vi "UHR-Fleezers Control (host) - 10.5.vi"() -> ()   [LabVIEW 2011] (continued)
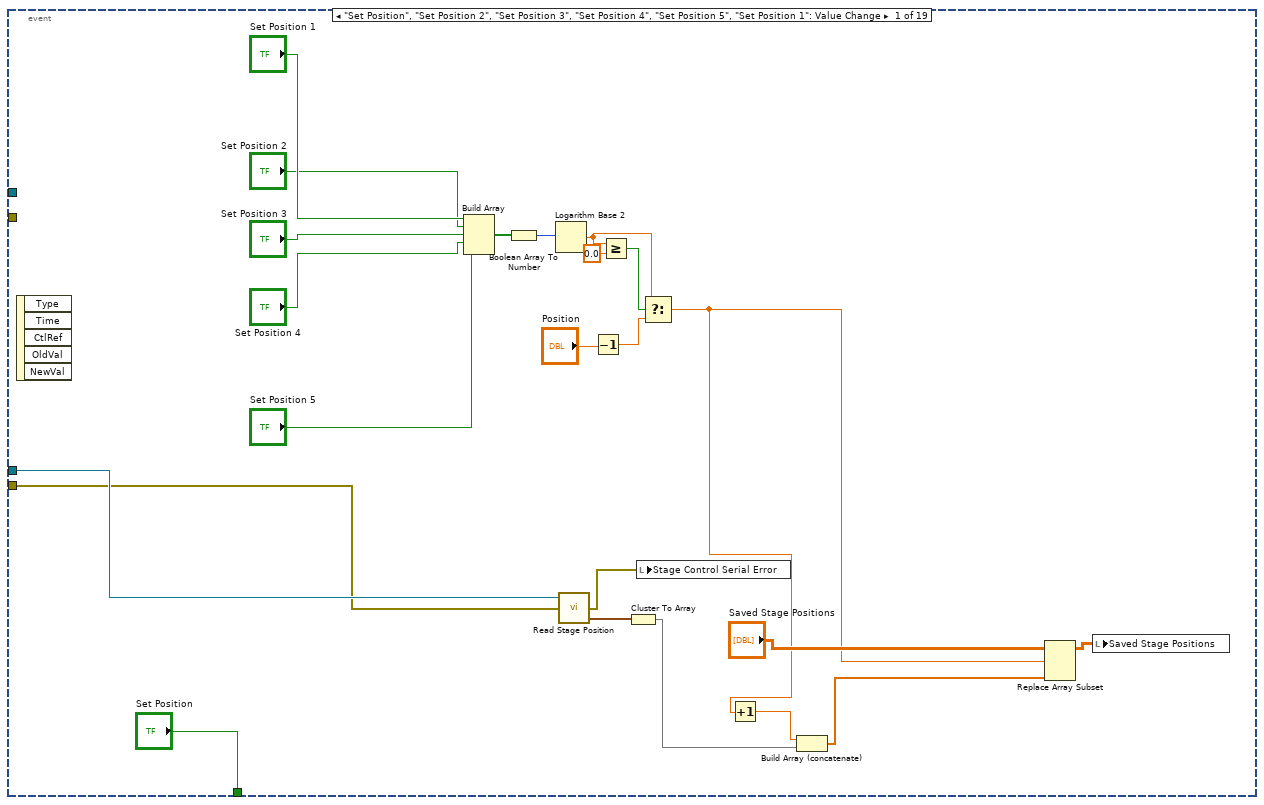
[diagram p2: hidden frame]
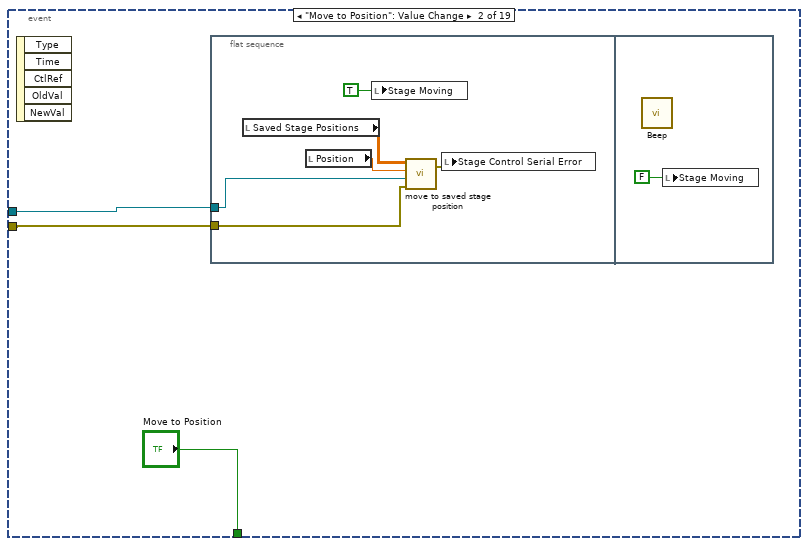
[diagram p3: hidden frame]
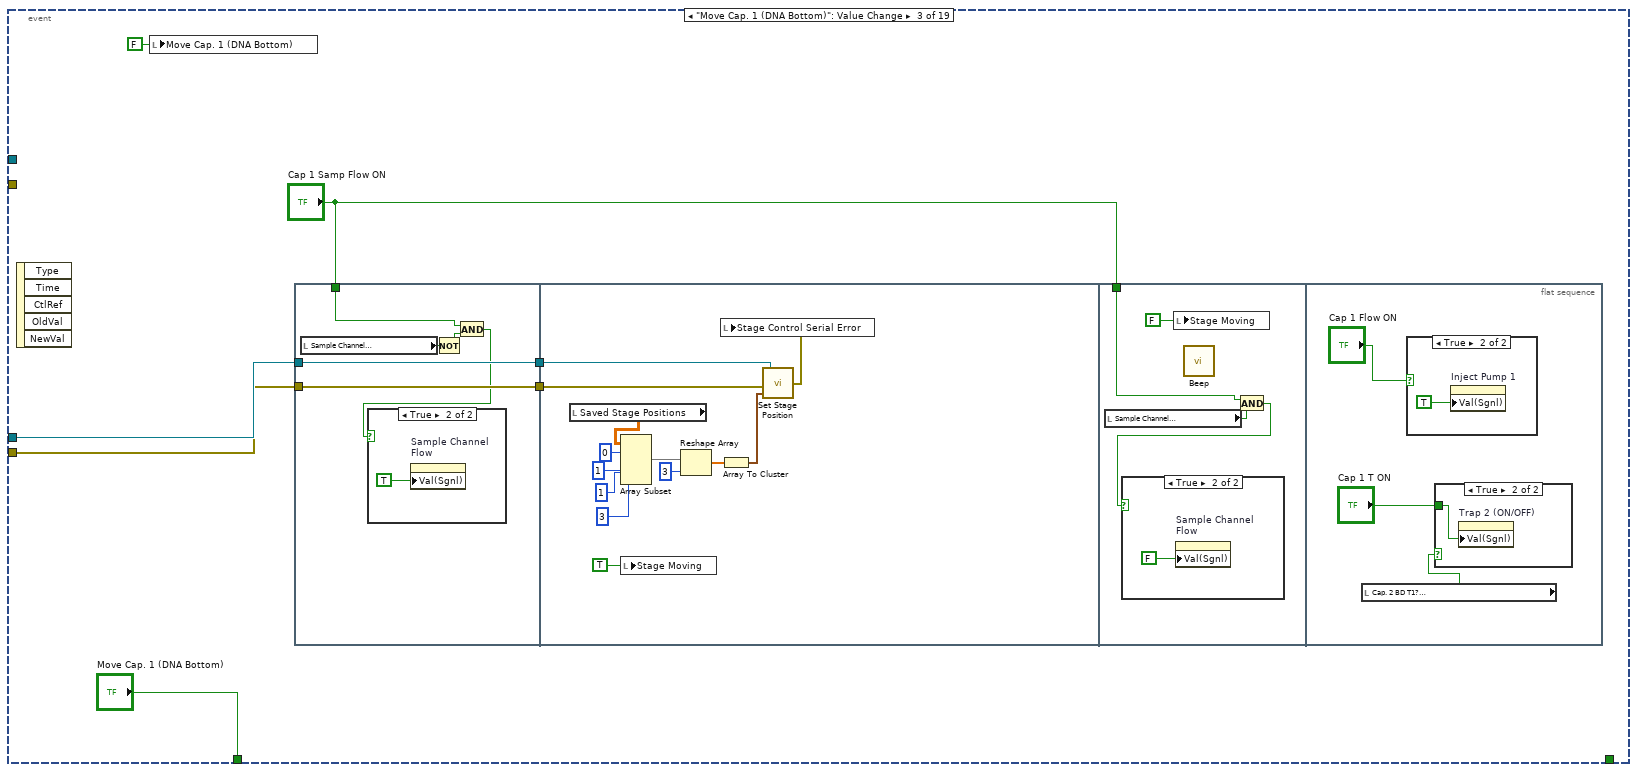
[diagram p4: hidden frame]
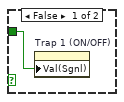
[diagram p8: hidden frame]
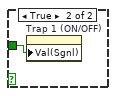
[diagram p12: hidden frame]
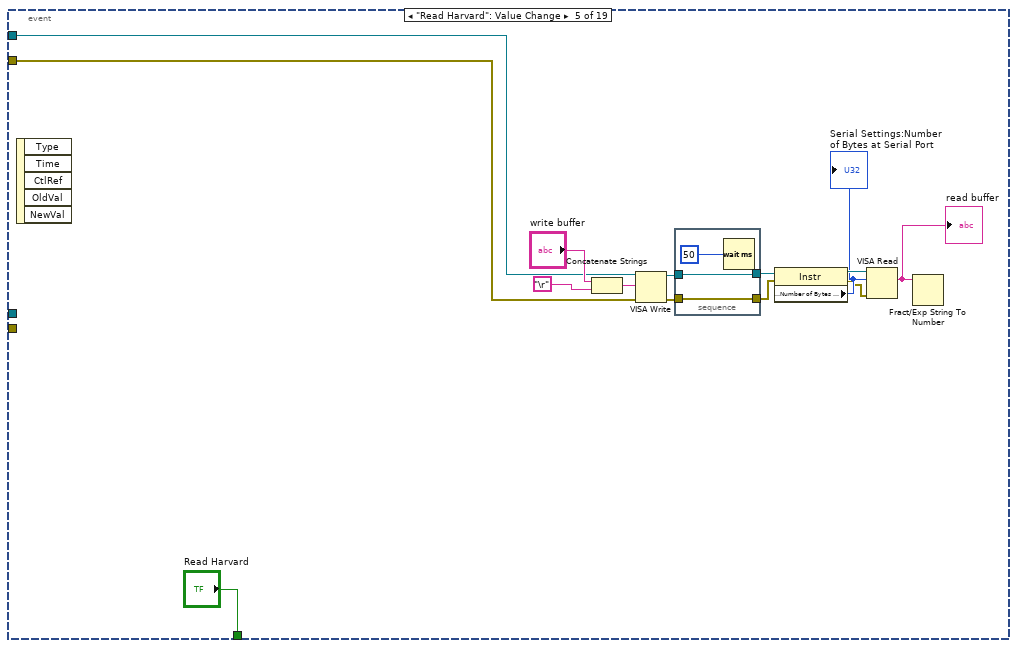
[diagram p13: hidden frame]
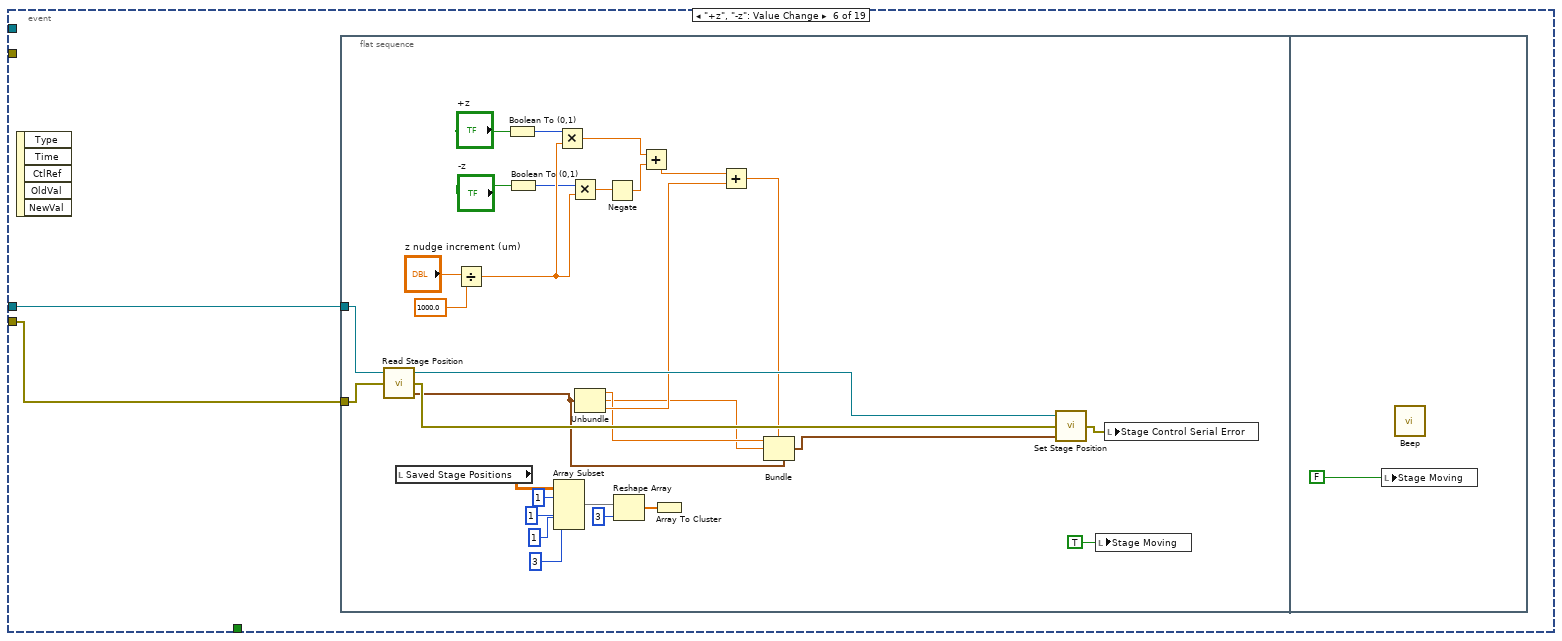
[diagram p14: hidden frame]
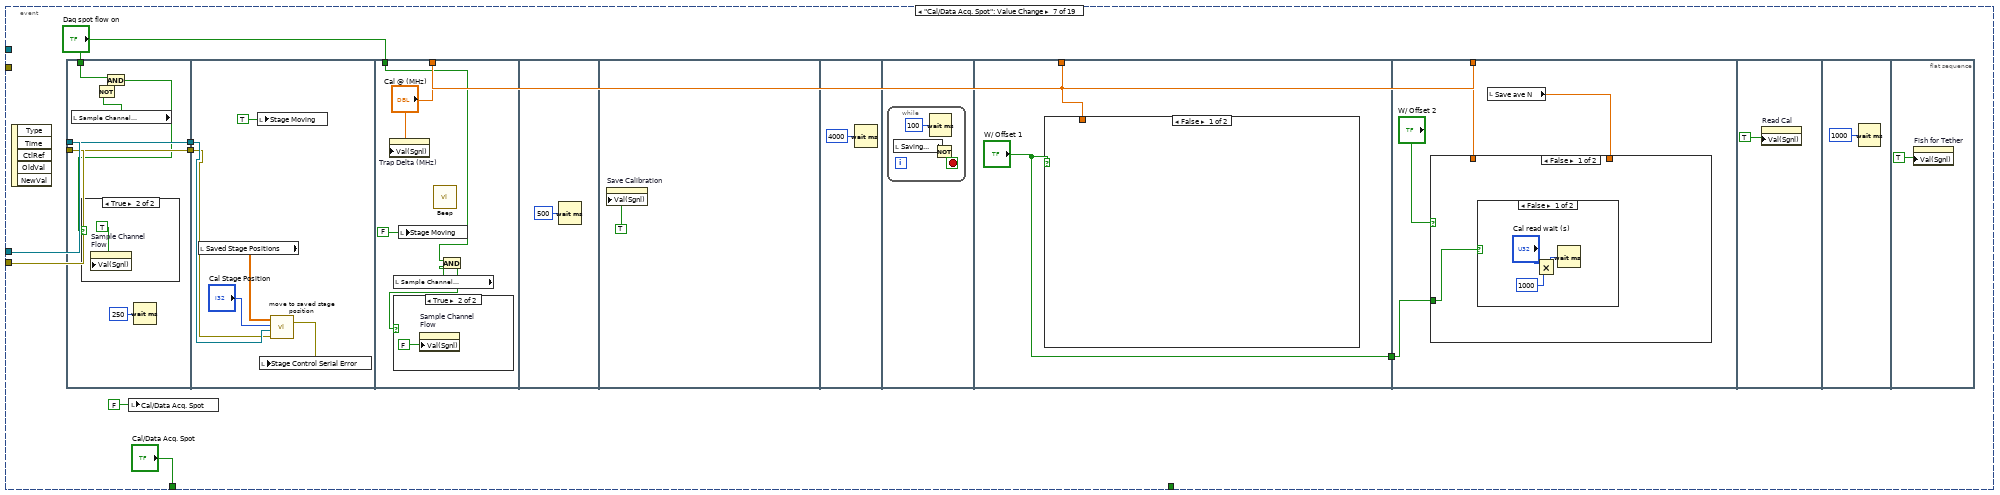
[diagram p15: hidden frame]
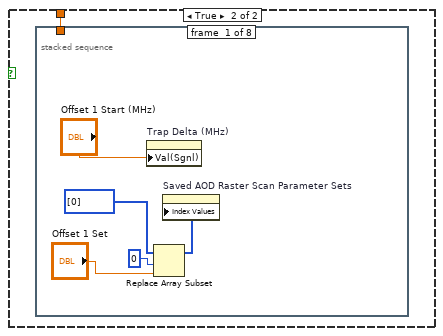
[diagram p18: hidden frame]
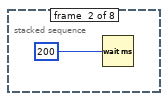
[diagram p19: hidden frame]
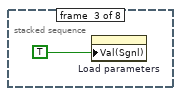
[diagram p20: hidden frame]
    n2214 = Subtract(x=w2595, y="Offset (nm)") -> (x-y=w2773:dbl[])
    n2215 = case shown="True" "Read Lateness and Rel Phase" {
      tunnel: w2615 -> [w3099 w3121]
      tunnel: w2614 -> [w3100 w3120]
      tunnel: [w3099 w3119] -> w2802
      tunnel: [w3100 w3118] -> w2801
      frame False {
      }
      frame True {
        n2216 = xnode "Read/Write Control"("FPGA VI Reference In"=w3121, "error in"=w3120) -> ("FPGA VI Reference Out"=w3119:T19, "error out"=w3118:errorcluster, "GI Relative phase"=→"GI relative phase":i16, "Relative phase"=→"Relative phase (AI1)":i16, "AI Late Counter"=→"Late Counter (AI1)":u16, "GI Late Counter"=→"GI Late Counter":u16, "MCL Late Counter"=→"MCL Late Counter":u16, "MCL Relative Phase"=→"Relative Phase (MCL)":i16, "APD Acq Relative Phase"=→"APD Acq Relative Phase":i16, "APD 1 Gate Relative Phase"=→"APD 1 Gate Relative Phase":i16, "APD 2 Gate Relative Phase"=→"APD 2 Gate Relative Phase":i16, "APD Acq Late Counter"=→"APD Acq Late Counter":u16, "APD 1 Gate Late Counter"=→"APD 1 Gate Late Counter":u16, "APD 2 Gate Late Counter"=→"APD 2 Gate Late Counter":u16, "Green FB Relative Phase"=→"Relative phase (Green FB)":i16, "GI Relative phase 2"=→"GI relative phase 2":i16, "GI Late Counter 2"=→"GI Late Counter 2":u16, "Trap Pos FIFO Timeout"=→"Trap Pos FIFO Timeout":u16, "Trap AI FIFO Timeout"=→"Trap AI FIFO Timeout":u16)
      }
    }
    n2217 = call <vilib>:"Mean.vi"("X"=w2775) -> ("mean"=w2601:dbl)  [unwired: 1 out]
    "T2 X" <- w2601
    n2218 = Negate(x=w2775) -> (-x=w2776:dbl[])
    n2219 = call <vilib>:"Mean.vi"("X"=w2599) -> ("mean"=w2602:dbl)  [unwired: 1 out]
    "T1 X" <- w2602
    n2220 = Negate(x=w2601) -> (-x=w2600:dbl)
    n2221 = Bundle By Name(cluster=w2808, "Y"=w2773) -> (w2747:waveform(dbl))
    "Bead Separation" <- w2747
    n2222 = Add(x=w2599, y=w2776) -> (x+y=w2777:dbl[])
    n2223 = Add(x=w2602, y=w2600) -> (x+y=w2824:dbl)
    n2224 = Subtract(x=w2602, y=w2600) -> (x-y=→"Difference":dbl)
    n2225 = Divide(x=w2777, y=2.0) -> (x/y=→"Vec Mean of T1 T2":dbl[])
    n2226 = Divide(x=w2824, y=2.0) -> (x/y=w2779:dbl)
    "Mean" <- w2779
    n2227 = feedback-in #21("Trap Trig. Fl.") -> ()
    n2228 = feedback #21("Trap Trig. Fl.") -> (w2633:bool)
    n2229 = And(x=w2635, y=w2633) -> (x .and. y?=w2634:bool)
    n2230 = case "If have just turned off triggering" shown="True" w2634 {
      tunnel: w2615 -> [_ w2934]
      tunnel: w2614 -> [_ w2933]
      frame False {
      }
      frame True {
        w2932 = FALSE ("FPGA Trap Trig")
        n2231 = xnode "Read/Write Control"("FPGA VI Reference In"=w2934, "error in"=w2933, "FPGA Trap Trig"=w2932) -> ("FPGA VI Reference Out"=w2931:T19, "error out"=w2930:errorcluster)
        n2232 = xnode "Read/Write Control"("FPGA VI Reference In"=w2931, "error in"=w2930, "TTrig?"=w2932) -> ()  [unwired: 2 out]
        n2233 = local write "Initializing"(FALSE ("Initializing")) -> ()
        n2234 = local write "Triggered"(FALSE ("Triggered")) -> ()
        n2235 = local write "Waiting"(FALSE ("Waiting")) -> ()
      }
    }
    n2236 = Not(x=w2633) -> (.not. x?=w2646:bool)
    n2237 = And(x="Trap Trig. Fl.", y=w2646) -> (x .and. y?=w2643:bool)
    n2238 = local read "Tether"() -> (w2780:bool)
    n2239 = Or(x=w2643, y="Reinitialize") -> (x .or. y?=w2629:bool)
    n2240 = feedback #22(w2639) -> (w2644:string)
    n2241 = Select(t=w2639, s=w2643, f=w2644) -> (s? t:f=w2638:string)
    n2242 = Select(t=w2639, s="Reinitialize", f=w2638) -> (s? t:f=w2637:string)
    n2243 = feedback #23(0) -> (w2641:i32)
    n2244 = feedback #24(w2773) -> (w2772:dbl[])
    n2245 = Build Array (concatenate)(w2773, w2772) -> (w2596:dbl[])
    n2246 = case "For determining if there is a tether still" shown="True" w2780 {
      tunnel: w2779 -> [_ w3058]
      frame False {
      }
      frame True {
        n2247 = Greater?(x="Lost Tether Alarm Threshold (pN)", y=w3058) -> (0:w3056:bool)
        n2248 = case shown="True" w3056 {
          frame False {
          }
          frame True {
            w3059 = FALSE ("Value (Signaling)")
            n2249 = flat-sequence {
              frame #0 {
                # "stop only if saving"
                n2250 = local read "Saving..."() -> (w3071:bool)
                n2251 = And(x=w3071, y="TA Cancel Save?") -> (x .and. y?=w3070:bool)
                n2252 = local write "Stop Saving"(w3070) -> ()
              }
              frame #1 {
                n2253 = case shown="True" "TA Green Off?" {
                  frame False {
                  }
                  frame True {
                    w3074 = FALSE ("Fl. Triggered...")
                    n2254 = local write "Fl. Triggered..."(w3074) -> ()
                    n2255 = property on="Green Laser ON/Interlacing" class="Bool (strict)"("Val(Sgnl)"=w3074) -> ()  [unwired: 2 in, 2 out]
                  }
                }
              }
            }
            n2256 = local read "Time tether formed"() -> (w3065:timestamp)
            n2257 = Get Date/Time In Seconds() -> (seconds since 1Jan1904=w3066:timestamp)
            n2258 = Subtract(x=w3066, y=w3065) -> (x-y=w3064:dbl)
            n2259 = Number To Decimal String(number=w3064) -> (decimal integer string=w3061:string)  [unwired: 1 out]
            n2260 = local read "Messages"() -> (w3068:string)
            n2261 = call <vilib>:"Beep.vi"() -> ()  [unwired: 3 in, 9 out]
            n2262 = Concatenate Strings("Lost tether (" ("Message to add"), w3061, " s)." ("string")) -> (w3063:string)
            n2263 = local write "Tether"(FALSE ("Tether")) -> ()
            n2264 = call "Update messages.vi"("Message to add"=w3063, "Old message string"=w3068) -> ("New message string"=w3067:string)
            n2265 = local write "Messages"(w3067) -> ()
            n2266 = local write "Dip for Protein"(w3059) -> ()
            n2267 = property on="Trap Pos. FB ON" class="Bool (strict)"("Val(Sgnl)"=w3059) -> ()  [unwired: 2 in, 2 out]
            n2268 = property on="Trap Trig. Fl." class="Bool (strict)"("Val(Sgnl)"=w3059) -> ()  [unwired: 2 in, 2 out]
          }
        }
      }
    }
    n2269 = case "For triggering actions based on the trap position (e.g., turning the excitation laser on if trap under feedback moves so far)" shown="True" "Trap Trig. Fl." {
      tunnel: w2624 -> [_ w2947]
      tunnel: w2637 -> [_ w2946]
      tunnel: ["" ("t") w2945] -> w2645
      tunnel: w2629 -> [_ w2944]
      tunnel: [0 ("t") w2943] -> w2642
      tunnel: w2641 -> [_ w2942]
      tunnel: w2615 -> [_ w2941]
      tunnel: w2614 -> [_ w2940]
      frame False {
      }
      frame True {
        n2270 = case shown="\"Initialize\", Default" w2946 {
          tunnel: w2947 -> [w2964 _ _ w3012]
          tunnel: [w2961 w2993 "" ("t") w3015] -> w2945
          tunnel: w2944 -> [_ _ _ w3003]
          tunnel: [w2960 w2990 0 ("t") w3004] -> w2943
          tunnel: w2942 -> [_ w2992 _ w3010]
          tunnel: w2941 -> [w2949 w2987 _ w3006]
          tunnel: w2940 -> [w2948 w2986 _ w3005]
          frame "Wait for trigger" {
            n2271 = local read "Trap Trig. (FPGA)"() -> (w2952:bool)
            n2272 = Subtract(x=w2964, y="Mean T1 Position\nto compare (nm)") -> (x-y=w2957:dbl[])
            n2273 = call <vilib>:"Std Deviation and Variance.vi"("X"=w2957) -> ("mean"=→"mean":dbl, "standard deviation"=→"standard\ndeviation":dbl)  [unwired: 1 in, 1 out]
            n2274 = Array Max & Min(array=w2957) -> (max value=→"max value":dbl, min value=→"min value":dbl)  [unwired: 2 out]
            n2275 = Greater?(x=w2957, y="Threshold (nm)") -> (0:w2967:bool[])
            n2276 = case shown="True" w2952 {
              tunnel: w2949 -> [_ w2973]
              tunnel: w2948 -> [_ w2972]
              tunnel: [FALSE ("TTrig?") w2971] -> w2955
              frame False {
              }
              frame True {
                n2277 = xnode "Read/Write Control"("FPGA VI Reference In"=w2973, "error in"=w2972) -> ("TTrig?"=w2971:bool)  [unwired: 2 out]
              }
            }
            n2278 = Or Array Elements(Boolean array=w2967) -> (logical OR=w2954:bool)
            n2279 = Select(t=w2955, s=w2952, f=w2954) -> (s? t:f=w2953:bool)
            n2280 = Not(x=w2952) -> (.not. x?=w2951:bool)
            n2281 = And(x=w2953, y=w2951) -> (x .and. y?=w2950:bool)
            n2282 = Select(t="Triggered", s=w2953, f="Wait for trigger") -> (s? t:f=w2961:string)
            n2283 = case shown="True" w2953 {
              tunnel: [0 0] -> w2960
              tunnel: w2949 -> [_ w2978]
              tunnel: w2948 -> [_ w2977]
              frame False {
                "Waiting" <- TRUE ("Waiting")
              }
              frame True {
                n2284 = xnode "Read/Write Control"("FPGA VI Reference In"=w2978, "error in"=w2977, "TTrig?"=FALSE) -> ()  [unwired: 2 out]
                n2285 = local read "Messages"() -> (w2981:string)
                n2286 = call <vilib>:"Beep.vi"() -> ()  [unwired: 12 in]
                n2287 = call "Update messages.vi"("Message to add"="Unwinding trigger.", "Old message string"=w2981) -> ("New message string"=w2982:string)
                n2288 = local write "Messages"(w2982) -> ()
                n2289 = local write "Waiting"(FALSE ("Waiting")) -> ()
                "Triggered" <- TRUE ("Triggered")
              }
            }
            n2290 = case "Only need to turn on laser if host triggered" shown="True" w2950 {
              frame False {
              }
              frame True {
                n2291 = property on="Green Laser ON/Interlacing" class="Bool (strict)"("Val(Sgnl)"=TRUE ("Value (Signaling)")) -> ()  [unwired: 2 in, 2 out]
              }
            }
          }
          frame "Triggered" {
            n2292 = local read "Trap Trig. (FPGA)"() -> (w2989:bool)
            n2293 = Increment(x=w2992) -> (x+1=w2990:i32)
            n2294 = Greater Or Equal?(x=w2990, y="Fl. ON time (n)") -> (x >= y?=w2988:bool)
            n2295 = Select(t="Wait for trigger", s=w2988, f="Triggered" ("t")) -> (s? t:f=w2993:string)
            n2296 = And(x=w2988, y=w2989) -> (x .and. y?=w2985:bool)
            n2297 = case shown="True" w2985 {
              tunnel: w2987 -> [_ w2997]
              tunnel: w2986 -> [_ w2996]
              frame False {
              }
              frame True {
                n2298 = xnode "Read/Write Control"("FPGA VI Reference In"=w2997, "error in"=w2996, "FPGA Trap Trig"=TRUE) -> ()  [unwired: 2 out]
              }
            }
            n2299 = case shown="True" w2988 {
              frame False {
              }
              frame True {
                w2999 = FALSE ("Value (Signaling)")
                n2300 = local write "Triggered"(w2999) -> ()
                n2301 = local write "Waiting"(TRUE ("Waiting")) -> ()
                n2302 = property on="Green Laser ON/Interlacing" class="Bool (strict)"("Val(Sgnl)"=w2999) -> ()  [unwired: 2 in, 2 out]
              }
            }
          }
          frame "Do nothing" {
          }
          frame "Initialize", Default {
            n2303 = Increment(x=w3010) -> (x+1=w3014:i32)
            n2304 = Select(t=1, s=w3003, f=w3014) -> (s? t:f=w3004:i32)
            n2305 = feedback #25(w3012) -> (w3018:dbl[])
            n2306 = Build Array (concatenate)(w3012, w3018) -> (w3011:dbl[])
            n2307 = Greater Or Equal?(x=w3004, y="Wait to get offset (n)") -> (x >= y?=w3007:bool)
            n2308 = Select(t=w3012, s=w3003, f=w3011) -> (s? t:f=w3013:dbl[])
            n2309 = feedback-in #25(w3013) -> ()
            n2310 = call <vilib>:"Mean.vi"("X"=w3013) -> ("mean"=w3008:dbl)  [unwired: 1 out]
            n2311 = local write "Mean T1 Position\nto compare (nm)"(w3008) -> ()
            n2312 = case shown="True" w3003 {
              tunnel: w3006 -> [_ w3024]
              tunnel: w3005 -> [_ w3023]
              frame False {
              }
              frame True {
                w3020 = FALSE ("FPGA Trap Trig")
                n2313 = xnode "Read/Write Control"("FPGA VI Reference In"=w3024, "error in"=w3023, "FPGA Trap Trig"=w3020) -> ("FPGA VI Reference Out"=w3022:T19, "error out"=w3021:errorcluster)
                n2314 = xnode "Read/Write Control"("FPGA VI Reference In"=w3022, "error in"=w3021, "TTrig?"=w3020) -> ()  [unwired: 2 out]
              }
            }
            n2315 = Select(t="Wait for trigger", s=w3007, f="Initialize") -> (s? t:f=w3015:string)
            n2316 = case shown="True" w3007 {
              tunnel: w3008 -> [_ w3027]
              tunnel: w3006 -> [_ w3036]
              tunnel: w3005 -> [_ w3035]
              frame False {
                n2317 = local write "Waiting"(FALSE ("Waiting")) -> ()
                "Initializing" <- TRUE ("Initializing")
              }
              frame True {
                n2318 = local read "Threshold (nm)"() -> (w3039:dbl)
                n2319 = local read "AOM X Cal (nm/MHz)"() -> (w3038:dbl)
                n2320 = Add(x=w3027, y=w3039) -> (x+y=w3040:dbl)
                n2321 = Divide(x=w3040, y=w3038) -> (x/y=w3037:dbl)
                n2322 = call "IR AOM freq to word.vi"("Frequency In (MHz)"=w3037) -> ("Frequency Word Out (double)"=w3034:dbl)
                n2323 = local write "Initializing"(FALSE ("Initializing")) -> ()
                n2324 = local write "Waiting"(TRUE ("Waiting")) -> ()
                n2325 = To Quad Integer(1:w3034) -> (0:w3033:i64)
                n2326 = xnode "Read/Write Control"("FPGA VI Reference In"=w3036, "error in"=w3035, "FPGA TTrig Thresh"=w3033) -> ("FPGA VI Reference Out"=w3030:T19, "error out"=w3029:errorcluster)
                n2327 = xnode "Read/Write Control"("FPGA VI Reference In"=w3030, "error in"=w3029, "FPGA Trap Trig"=TRUE) -> ()  [unwired: 2 out]
              }
            }
          }
        }
      }
    }
    n2328 = feedback-in #22(w2645) -> ()
    n2329 = feedback-in #23(w2642) -> ()
    n2330 = Split 1D Array(array=w2596, index=w2659) -> (first subarray=w2769:dbl[])  [unwired: 1 out]
    n2331 = feedback-in #24(w2769) -> ()
    n2332 = call <vilib>:"Mean.vi"("X"=w2769) -> ("mean"=w2768:dbl)  [unwired: 1 out]
    "Bead Mean (nm)" <- w2768
    n2333 = Subtract(x=w2769, y=w2768) -> (x-y=w2767:dbl[])
    n2334 = Square(x=w2767) -> (x^2=w2766:dbl[])
    n2335 = call <vilib>:"Mean.vi"("X"=w2766) -> ("mean"=w2765:dbl)  [unwired: 1 out]
    n2336 = Square Root(x=w2765) -> (sqrt(x)=w2764:dbl)
    n2337 = Multiply(x=10.0, y=w2764) -> (x*y=→"RMS (Ang)":dbl)
    n2338 = xnode "Read/Write Control"("FPGA VI Reference In"=w2802, "error in"=w2801) -> ("FPGA VI Reference Out"=w2627:T19, "error out"=w2626:errorcluster, "AI2 Y Sum Set 1"=w2908:i16, "AI2 Y Sum Set 2"=w2907:i16, "AI1 X Set 1"=w2691:fxp<+/-,16,1>, "AI1 X Set 2"=w2690:fxp<+/-,16,1>, "Trap Pos FB Int Signal"=→"Trap Pos FB Int Signal":fxp<+/-,24,9>, "Trap Pos FB Int-Norm Signal"=→"Trap Pos FB Int-Norm Signal":fxp<+/-,16,1>, "Trap Pos FB Action"=w2684:i64, "Scanning"=→"AOD Scanning":bool, "Scan I"=→"AOD Scan I":u64, "Scanning MCL"=w2910:bool, "Scan I (MCL)"=→"MCL Scan I":u64, "Green FB Signals"=w2847:T46, "TTrig Sig"=w2613:i64, "TTrig Fin Thresh"=w2609:i64)
    "MCL Scanning" <- w2910
    "Trap Pos FB Action" <- w2684
    n2339 = local read "FB Trig Integrate"() -> (w2607:u32)
    n2340 = Divide(x=w2613, y=w2607) -> (x/y=w2606:dbl)
    "TTrig Sig (Int)" <- w2606
    n2341 = Divide(x=w2609, y=w2607) -> (x/y=w2604:dbl)
    "TTrig Fin Thresh (Int)" <- w2604
    n2342 = local read "AOM X Cal (nm/MHz)"() -> (w2612:dbl)
    n2343 = local read "AI2 (V)"() -> (w2909:cluster{"Set 1":dbl, "Set 2":dbl})
    n2344 = Bundle By Name(cluster=w2909, "Set 1"=w2908, "Set 2"=w2907) -> (w2905:cluster{"Set 1":dbl, "Set 2":dbl})
    n2345 = Divide(x=w2684, y=327.67) -> (x/y=→"Action (%)":dbl)
    n2346 = local read "Trap X (AI1)"() -> (w2704:T10)
    n2347 = call "IR AOM word double to freq.vi"("Frequency Word In (double)"=w2604) -> ("Frequency Out (MHz)"=w2603:dbl)
    n2348 = call "IR AOM word double to freq.vi"("Frequency Word In (double)"=w2606) -> ("Frequency Out (MHz)"=w2605:dbl)
    n2349 = Divide(x=w2905, y=3276.7) -> (x/y=w2904:cluster{"Set 1":dbl, "Set 2":dbl})
    n2350 = Multiply(x=w2605, y=w2612) -> (x*y=w2611:dbl)
    "TTrig Sig (nm)" <- w2611
    n2351 = Multiply(x=w2603, y=w2612) -> (x*y=w2610:dbl)
    "TTrig Fin Thresh (nm)" <- w2610
    n2352 = local write "AI2 (V)"(w2904) -> ()
    n2353 = Bundle(cluster=w2704, "Trap 1"=w2691, "Trap 2"=w2690) -> (→"Trap X (AI1)":T10)
    n2354 = Bundle(w2611, w2610) -> (→"TTrig":cluster{dbl, dbl})  [unwired: 1 in]
    n2355 = Divide(x=w2847, y=3276.7) -> (x/y=w2843:T47)
    n2356 = Unbundle By Name(w2843) -> ("Green FB Ch 0"=w2846:dbl, "Green FB Ch 1"=w2845:dbl, "Green FB Ch 2"=w2844:dbl)
    n2357 = Divide(x=w2846, y=w2844) -> (x/y=w2842:dbl)
    n2358 = Divide(x=w2845, y=w2844) -> (x/y=w2841:dbl)
    n2359 = flat-sequence "To save data" {
      tunnel: [w3895] -> w2928
      tunnel: [w3896] -> w2927
      tunnel: w2878 -> [w3889]
      tunnel: w2632 -> [w3893]
      tunnel: ["Save Calibration"] -> w2901
      tunnel: w2898 -> [w3892]
      tunnel: [w3885] -> w2897
      tunnel: [w3882] -> w2896
      tunnel: [w3879] -> w2895
      tunnel: w2877 -> [w3881]
      tunnel: w2784 -> [w3875]
      tunnel: [w3875] -> w2783
      tunnel: ["Start Saving"] -> w2749
      tunnel: [w3869] -> w2672
      tunnel: [w3868] -> w2671
      tunnel: w2928 -> [w4130]
      tunnel: w2927 -> [w4129]
      tunnel: w2673 -> [w4128]
      tunnel: w2901 -> [w4127]
      tunnel: w2897 -> [w4125]
      tunnel: w2896 -> [w4124]
      tunnel: w2895 -> [w4123]
      tunnel: w2758 -> [w4122]
      tunnel: w2794 -> [w4121]
      tunnel: w2783 -> [w4120]
      tunnel: w2749 -> [w4119]
      tunnel: w2747 -> [w4118]
      tunnel: w2723 -> [w4117]
      tunnel: w2672 -> [w4116]
      tunnel: w2671 -> [w4115]
      tunnel: w2670 -> [w4114]
      frame #0 {
        n2360 = Or(x="Save N Sets", y="Start Saving") -> (x .or. y?=w3876:bool)
        n2361 = To Double Precision Float(number=w3892) -> (double precision float=w3886:dbl)
        n2362 = Build Array(w3876, "Save Calibration", w3889, w3881) -> (w3891:bool[])
        n2363 = Compound Arithmetic op=OR("Save Calibration", w3889, w3876, w3881) -> (w3894:bool)
        n2364 = Boolean Array To Number(Boolean array=w3891) -> (number=w3888:u32)
        n2365 = feedback #26(FALSE ("Save APD Data\nwith Trap Data")) -> (w3870:bool)
        n2366 = feedback #27(refnum<k0> refnum) -> (w3897:refnum<file>)
        n2367 = feedback #28(refnum<k0> refnum) -> (w3872:refnum<file>)
        n2368 = feedback #29(FALSE ("Save APD Data\nwith Trap Data")) -> (w3880:bool)
        n2369 = feedback #30(refnum<k0> refnum) -> (w3883:refnum<file>)
        n2370 = feedback #31(0) -> (w3899:i32)
        n2371 = feedback #32() -> (w3887:u32)  [unwired: 1 out]
        n2372 = case shown="True" w3894 {
          tunnel: [w3906 1] -> w3895
          tunnel: w3899 -> [w3908 _]
          tunnel: [w3907 w3926] -> w3896
          tunnel: w3897 -> [w3907 _]
          tunnel: w3893 -> [_ w3946]
          tunnel: w3886 -> [_ w3944]
          tunnel: w3888 -> [_ w3947]
          tunnel: [w3905 w3925] -> w3885
          tunnel: w3887 -> [w3905 _]
          tunnel: [w3904 w3923] -> w3882
          tunnel: w3883 -> [w3904 _]
          tunnel: [w3903 w3922] -> w3879
          tunnel: w3880 -> [w3903 _]
          tunnel: "Start Saving" -> [_ w3920]
          tunnel: w3875 -> [_ w3919]
          tunnel: [w3902 w3910] -> w3868
          tunnel: w3872 -> [w3902 _]
          tunnel: [w3901 w3909] -> w3869
          tunnel: w3870 -> [w3901 _]
          frame False {
            n2373 = Increment(x=w3908) -> (x+1=w3906:i32)
          }
          frame True {
            w3916 = FALSE ("Start Saving")
            w3921 = 9.0  # File Version
            w3929 = FALSE ("prepend array or string size? (T)")
            w3927 = T24."big-endian, network order" ("byte order (0:big-endian, network order)")
            n2374 = local read "BD 1 Frequency 1 (MHz)"() -> (w3943:dbl)
            n2375 = local read "BD 2 Frequency 1 (MHz)"() -> (w3942:dbl)
            n2376 = local read "BD 1 Frequency 2 (MHz)"() -> (w3941:dbl)
            n2377 = local read "BD 2 Frequency 2 (MHz)"() -> (w3940:dbl)
            n2378 = local read "BD 1 Frequency 3 (MHz)"() -> (w3939:dbl)
            n2379 = local read "BD 2 Frequency 3 (MHz)"() -> (w3938:dbl)
            n2380 = Array Size(array=w3919) -> (size(s)=w3918:i32)
            n2381 = To Double Precision Float(number=w3918) -> (double precision float=w3917:dbl)
            n2382 = local write "Save Calibration"(w3916) -> ()
            n2383 = local write "Start Saving"(w3916) -> ()
            n2384 = Build Array("Save APD Data\nwith Trap Data", "Save Trap Pos. Data") -> (w3913:bool[])
            n2385 = Boolean Array To Number(Boolean array=w3913) -> (number=w3912:u32)
            n2386 = Build Array(w3943, w3942, w3941, w3940, w3939, w3938) -> (w3937:dbl[])
            n2387 = case shown="4" w3947 {
              tunnel: w3946 -> [w4018 w4038 w4054 w4092]
              tunnel: w3917 -> [w4023 w4045 w4074 w4111]
              tunnel: w3944 -> [w4022 w4044 w4073 w4110]
              tunnel: [w4019 w4040 w4065 w4102] -> w3935
              tunnel: [w4010 "Cal sets to save" w4055 w4093] -> w3925
              tunnel: w3937 -> [w4020 w4041 w4067 w4104]
              tunnel: "Save APD Data\nwith Trap Data" -> [w4017 _ w4051 w4090]
              tunnel: [w4017 w4032 w4051 w4090] -> w3922
              tunnel: w3921 -> [w4013 w4033 w4049 w4088]
              tunnel: w3920 -> [w4012 _ _ _]
              tunnel: [w4003 w4032 w4048 w4078] -> w3909
              tunnel: "Save Trap Pos. Data" -> [w4003 _ w4048 w4078]
              tunnel: w3912 -> [w4002 _ w4047 w4077]
              frame 1, Default {
                # "timeseries"
                n2388 = case shown="True" "Profile" {
                  tunnel: [w4026 w4030] -> w4007
                  tunnel: [w4026 w4029] -> w4006
                  tunnel: [w4026 w4028] -> w4005
                  tunnel: [w4026 w4027] -> w4004
                  frame False {
                    w4026 = 0.0 ("f")
                  }
                  frame True {
                    n2389 = local read "Current Position"() -> (w4031:cluster{dbl, dbl, dbl})
                    n2390 = local read "Y change (mm)"() -> (w4027:dbl)
                    n2391 = Unbundle(w4031) -> (w4030:dbl, w4029:dbl, w4028:dbl)
                  }
                }
                n2392 = local read "Save ave N"() -> (w4025:dbl)
                n2393 = Multiply(x=w4025, y=w4018) -> (x*y=w4024:dbl)
                n2394 = To Double Precision Float(number=w4002) -> (double precision float=w4016:dbl)
                n2395 = Build Array(w4013, w4018, w4024, w4023, w4022, 0.0 ("f")) -> (w4021:dbl[])
                n2396 = Build Array(w4016, w4007, w4006, w4005, w4004) -> (w4014:dbl[])
                n2397 = Select(t=u32 4000000000, s=w4012, f="N sets to save") -> (s? t:f=w4010:u32)
                n2398 = Build Array (concatenate)(w4021, w4020, w4014) -> (w4019:dbl[])
              }
              frame 2 {
                w4035 = 0.0 ("f")
                w4032 = FALSE ("Save APD Data\nwith Trap Data")
                # "calibration"
                n2399 = Boolean To (0,1)(Boolean=w4032) -> (0, 1=w4037:i16)
                n2400 = To Double Precision Float(number=w4037) -> (double precision float=w4036:dbl)
                n2401 = Build Array(w4036, w4035, w4035, w4035, w4035) -> (w4034:dbl[])
                n2402 = Build Array(w4033, w4038, w4038, w4045, w4044, 1.0 ("t")) -> (w4042:dbl[])
                n2403 = Build Array (concatenate)(w4042, w4041, w4034) -> (w4040:dbl[])
                "Calibrating Trap..." <- TRUE ("Calibrating...")
              }
              frame 4 {
                w4052 = 0.0 ("f")
                # "scan dir (x/y = 0/1)"
                # "cycles/step"
                # "n scans (f/b)"
                # "steps"
                # "freq. range"
                # "AOD raster scan"
                n2404 = local read "Number of F/B Scans (AOD)"() -> (w4059:u16)
                n2405 = local read "Cycles/step (AOD)"() -> (w4061:u64)
                n2406 = local read "Scan Range (MHz)"() -> (w4064:dbl)
                n2407 = local read "Scan steps (AOD)"() -> (w4063:u64)
                n2408 = local read "Scan BD"() -> (w4071:bool)
                n2409 = local read "Save ave N"() -> (w4076:dbl)
                n2410 = Boolean To (0,1)(Boolean=w4071) -> (0, 1=w4070:i16)
                n2411 = To Double Precision Float(number=w4059) -> (double precision float=w4058:dbl)
                n2412 = To Double Precision Float(number=w4063) -> (double precision float=w4062:dbl)
                n2413 = To Double Precision Float(number=w4061) -> (double precision float=w4060:dbl)
                n2414 = To Double Precision Float(number=w4070) -> (double precision float=w4069:dbl)
                n2415 = Multiply(x=w4076, y=w4054) -> (x*y=w4075:dbl)
                n2416 = To Double Precision Float(number=w4047) -> (double precision float=w4053:dbl)
                n2417 = Build Array(w4053, w4052, w4052, w4052, w4052) -> (w4050:dbl[])
                n2418 = local read "N sets should be saved"() -> (w4056:dbl)
                n2419 = Build Array(w4069, w4064, w4062, w4060, w4058) -> (w4066:dbl[])
                n2420 = Build Array(w4049, w4054, w4075, w4074, w4073, 2.0 ("t")) -> (w4068:dbl[])
                n2421 = Round Toward +Infinity(x=w4056) -> (ceil(x): smallest int >= x=w4057:dbl)
                n2422 = Build Array (concatenate)(w4068, w4067, w4050, w4066) -> (w4065:dbl[])
                n2423 = To Unsigned Long Integer(number=w4057) -> (unsigned 32bit integer=w4055:u32)
              }
              frame 8 {
                w4085 = 0.0 ("f")
                # "MCL raster scan"
                n2424 = local read "Number of scans (MCL)"() -> (w4080:u64)
                n2425 = local read "Scan lines (y)"() -> (w4079:u64)
                n2426 = local read "2D or 1D Scan"() -> (w4082:bool)
                n2427 = local read "Scan Range (V)\n(of steps)"() -> (w4101:dbl)
                n2428 = local read "Fast Scan Dir"() -> (w4108:bool)
                n2429 = local read "Cycles/step (MCL)"() -> (w4098:u64)
                n2430 = local read "Scan steps (MCL)"() -> (w4100:u64)
                n2431 = Select(t=w4079, s=w4082, f=w4080) -> (s? t:f=w4081:u64)
                n2432 = Boolean To (0,1)(Boolean=w4082) -> (0, 1=w4084:i16)
                n2433 = local read "Save ave N"() -> (w4113:dbl)
                n2434 = local read "Initial X"() -> (w4087:dbl)
                n2435 = local read "Initial Y"() -> (w4086:dbl)
                n2436 = To Double Precision Float(number=w4084) -> (double precision float=w4083:dbl)
                n2437 = Boolean To (0,1)(Boolean=w4108) -> (0, 1=w4107:i16)
                n2438 = To Double Precision Float(number=w4081) -> (double precision float=w4096:dbl)
                n2439 = To Double Precision Float(number=w4100) -> (double precision float=w4099:dbl)
                n2440 = To Double Precision Float(number=w4098) -> (double precision float=w4097:dbl)
                n2441 = To Double Precision Float(number=w4107) -> (double precision float=w4106:dbl)
                n2442 = Multiply(x=w4113, y=w4092) -> (x*y=w4112:dbl)
                n2443 = To Double Precision Float(number=w4077) -> (double precision float=w4091:dbl)
                n2444 = local read "N sets should be saved (MCL)"() -> (w4094:dbl)
                n2445 = Build Array(w4091, w4083, w4085, w4085, w4085) -> (w4089:dbl[])
                n2446 = Build Array(w4106, w4101, w4099, w4097, w4096, w4087, w4086) -> (w4103:dbl[])
                n2447 = Build Array(w4088, w4092, w4112, w4111, w4110, 3.0 ("t")) -> (w4105:dbl[])
                n2448 = Round Toward +Infinity(x=w4094) -> (ceil(x): smallest int >= x=w4095:dbl)
                n2449 = Build Array (concatenate)(w4105, w4104, w4089, w4103) -> (w4102:dbl[])
                n2450 = To Unsigned Long Integer(number=w4095) -> (unsigned 32bit integer=w4093:u32)
              }
            }
            n2451 = local read "Index"() -> (w3952:dbl)
            n2452 = call "Create new save file.vi"("Insert"="", "Ext"=".dat", "Index In"=w3952) -> ("Path Out"=w3911:path, "Index Out"=w3924:dbl)
            n2453 = local write "Save file name"(w3911) -> ()
            n2454 = local write "Index"(w3924) -> ()
            n2455 = local write "Save index"(w3924) -> ()
            n2456 = Array Size(array=w3935) -> (size(s)=w3936:i32)
            n2457 = Open/Create/Replace File(file path (use dialog)=w3911, operation (0:open)=T25."create", access (0:read/write)=enum16{"read/write", "read-only", "write-only"}."write-only") -> (refnum out=w3949:refnum<file>)  [unwired: 1 in, 4 out]
            n2458 = local write "Saving..."(TRUE ("Saving...")) -> ()
            n2459 = To Double Precision Float(number=w3936) -> (double precision float=w3934:dbl)
            n2460 = String Length(string="Comment (data description)") -> (length=w3932:i32)
            n2461 = To Double Precision Float(number=w3932) -> (double precision float=w3931:dbl)
            n2462 = Deny Access(7:w3949) -> (3:w3948:refnum<file>)  [unwired: 1 in, 2 out]
            n2463 = Build Array (concatenate)(w3934, w3935, w3931) -> (w3933:dbl[])
            n2464 = case "If fluorescence data to be saved" shown="True" w3922 {
              tunnel: w3911 -> [_ w4001]
              tunnel: [refnum<k0> refnum w3981] -> w3923
              frame False {
              }
              frame True {
                w3980 = 0.0
                n2465 = local read "APD Integration Time (s)"() -> (w3986:dbl)
                n2466 = local read "N APD Samp/step"() -> (w3979:dbl)
                n2467 = Path To String(path=w4001) -> (string=w4000:string)
                n2468 = String Length(string=w4000) -> (length=w3999:i32)
                n2469 = Subtract(x=w3999, y=4) -> (x-y=w3997:i32)
                n2470 = String Subset(string=w4000, length (rest)=w3997) -> (substring=w3996:string)  [unwired: 1 out]
                n2471 = Build Array(w3986, w3979, w3980, w3980, w3980, w3980, w3980, w3980) -> (w3983:dbl[])
                n2472 = Concatenate Strings(w3996, "_fl.dat" ("string")) -> (w3994:string)
                n2473 = Array Size(array=w3983) -> (size(s)=w3985:i32)
                n2474 = String To Path(string=w3994) -> (path=w3990:path)
                n2475 = Open/Create/Replace File(file path (use dialog)=w3990, operation (0:open)=T25."create", access (0:read/write)=enum16{"read/write", "read-only", "write-only"}."write-only") -> (refnum out=w3991:refnum<file>)  [unwired: 1 in, 4 out]
                n2476 = Deny Access(7:w3991) -> (3:w3987:refnum<file>)  [unwired: 1 in, 2 out]
                n2477 = To Double Precision Float(number=w3985) -> (double precision float=w3984:dbl)
                n2478 = Build Array (concatenate)(w3984, w3983) -> (w3982:dbl[])
                n2479 = Write to Binary File(file (use dialog)=w3987, data=w3982, 5:FALSE ("prepend array or string size? (T)"), 9:T24."big-endian, network order" ("byte order (0:big-endian, network order)")) -> (refnum out=w3981:refnum<file>)  [unwired: 1 in, 3 out]
              }
            }
            n2480 = case shown="True" w3909 {
              tunnel: w3911 -> [_ w3963]
              tunnel: [refnum<k0> refnum w3962] -> w3910
              frame False {
              }
              frame True {
                w3958 = 0.0 ("element")
                n2481 = Path To String(path=w3963) -> (string=w3977:string)
                n2482 = Build Array(w3958, w3958, w3958, w3958, w3958, w3958, w3958, w3958) -> (w3959:dbl[])
                n2483 = String Length(string=w3977) -> (length=w3976:i32)
                n2484 = Subtract(x=w3976, y=4) -> (x-y=w3974:i32)
                n2485 = Array Size(array=w3959) -> (size(s)=w3961:i32)
                n2486 = String Subset(string=w3977, length (rest)=w3974) -> (substring=w3973:string)  [unwired: 1 out]
                n2487 = To Double Precision Float(number=w3961) -> (double precision float=w3960:dbl)
                n2488 = Concatenate Strings(w3973, "_pos.dat" ("string")) -> (w3971:string)
                n2489 = Build Array (concatenate)(w3960, w3959) -> (w3957:dbl[])
                n2490 = String To Path(string=w3971) -> (path=w3967:path)
                n2491 = Open/Create/Replace File(file path (use dialog)=w3967, operation (0:open)=T25."create", access (0:read/write)=enum16{"read/write", "read-only", "write-only"}."write-only") -> (refnum out=w3968:refnum<file>)  [unwired: 1 in, 4 out]
                n2492 = Deny Access(7:w3968) -> (3:w3964:refnum<file>)  [unwired: 1 in, 2 out]
                n2493 = Write to Binary File(file (use dialog)=w3964, data=w3957, 5:FALSE ("prepend array or string size? (T)"), 9:T24."big-endian, network order" ("byte order (0:big-endian, network order)")) -> (refnum out=w3962:refnum<file>)  [unwired: 1 in, 3 out]
              }
            }
            n2494 = Write to Binary File(file (use dialog)=w3948, data=w3933, 5:w3929, 9:w3927) -> (refnum out=w3930:refnum<file>)  [unwired: 1 in, 3 out]
            n2495 = Write to Binary File(file (use dialog)=w3930, data="Comment (data description)", 5:w3929, 9:w3927) -> (refnum out=w3926:refnum<file>)  [unwired: 1 in, 3 out]
          }
        }
        n2496 = feedback-in #26(w3869) -> ()
        n2497 = feedback-in #27(w3896) -> ()
        n2498 = feedback-in #28(w3868) -> ()
        n2499 = feedback-in #29(w3879) -> ()
        n2500 = feedback-in #30(w3882) -> ()
        n2501 = feedback-in #31(w3895) -> ()
        n2502 = feedback-in #32(w3885) -> ()
      }
      frame #1 {
        n2503 = local read "Saving..."() -> (w4126:bool)
        n2504 = case shown="True" w4126 {
          tunnel: w4130 -> [_ w4140]
          tunnel: w4129 -> [_ w4154]
          tunnel: w4128 -> [_ w4150]
          tunnel: w4127 -> [_ w4149]
          tunnel: w4125 -> [_ w4148]
          tunnel: w4124 -> [_ w4143]
          tunnel: w4123 -> [_ w4142]
          tunnel: w4122 -> [_ w4141]
          tunnel: w4121 -> [_ w4139]
          tunnel: w4120 -> [_ w4137]
          tunnel: w4119 -> [_ w4136]
          tunnel: w4118 -> [_ w4135]
          tunnel: w4117 -> [_ w4134]
          tunnel: w4116 -> [_ w4133]
          tunnel: w4115 -> [_ w4132]
          tunnel: w4114 -> [_ w4131]
          frame False {
          }
          frame True {
            n2505 = Multiply(x=w4140, y=w4139) -> (x*y=→"Time (s)":dbl)
            n2506 = Less Or Equal?(x=w4140, y=w4148) -> (x <= y?=w4152:bool)
            n2507 = Or(x="Stop Saving", y="Abort save 2") -> (x .or. y?=w4144:bool)
            n2508 = Not(x=w4144) -> (.not. x?=w4153:bool)
            n2509 = And(x=w4152, y=w4153) -> (x .and. y?=w4151:bool)
            n2510 = case shown="True" w4151 {
              tunnel: w4154 -> [w4161 w4229]
              tunnel: [0.0 w4232] -> w4147
              tunnel: w4140 -> [_ w4230]
              tunnel: w4148 -> [_ w4231]
              tunnel: w4150 -> [_ w4226]
              tunnel: w4149 -> [_ _]
              tunnel: w4143 -> [w4159 w4219]
              tunnel: w4142 -> [w4158 w4220]
              tunnel: w4141 -> [_ w4218]
              tunnel: w4137 -> [_ w4217]
              tunnel: w4136 -> [_ w4171]
              tunnel: w4135 -> [_ w4210]
              tunnel: w4134 -> [_ w4188]
              tunnel: w4133 -> [w4155 w4169]
              tunnel: w4132 -> [w4156 w4168]
              tunnel: w4131 -> [_ w4165]
              frame False {
                w4157 = FALSE
                n2511 = Close File(refnum=w4161) -> ()  [unwired: 1 in, 2 out]
                n2512 = case shown="True" w4158 {
                  tunnel: w4159 -> [_ w4163]
                  frame False {
                  }
                  frame True {
                    n2513 = Close File(refnum=w4163) -> ()  [unwired: 1 in, 2 out]
                  }
                }
                n2514 = case shown="True" w4155 {
                  tunnel: w4156 -> [_ w4162]
                  frame False {
                  }
                  frame True {
                    n2515 = Close File(refnum=w4162) -> ()  [unwired: 1 in, 2 out]
                  }
                }
                n2516 = local write "Raster Scanning..."(w4157) -> ()
                n2517 = local write "Calibrating Trap..."(w4157) -> ()
                n2518 = call <vilib>:"Beep.vi"() -> ()  [unwired: 3 in, 9 out]
                n2519 = local write "Stop Saving"(w4157) -> ()
                "Saving..." <- w4157
              }
              frame True {
                n2520 = local read "Calibrating Trap..."() -> (w4221:bool)
                n2521 = case "Write fl. data" shown="True" w4220 {
                  tunnel: w4219 -> [_ w4255]
                  tunnel: w4218 -> [_ w4254]
                  frame False {
                  }
                  frame True {
                    n2522 = Write to Binary File(file (use dialog)=w4255, data=w4254, 5:FALSE ("prepend array or string size? (T)"), 9:T24."big-endian, network order" ("byte order (0:big-endian, network order)")) -> ()  [unwired: 1 in, 4 out]
                  }
                }
                n2523 = Greater?(x="Save ave N", y=1.0) -> (0:w4224:bool)
                n2524 = Not(x=w4221) -> (.not. x?=w4223:bool)
                n2525 = And(x=w4223, y=w4224) -> (x .and. y?=w4166:bool)
                n2526 = case shown="True" w4166 {
                  tunnel: w4165 -> [w4235 w4246]
                  tunnel: [w4235 w4238] -> w4164
                  tunnel: "Save ave N" -> [_ w4239]
                  frame False {
                  }
                  frame True {
                    w4236 = 2 ("dimension size")
                    n2527 = Array Size(array=w4246) -> (size(s)=w4240:i32)
                    n2528 = Divide(x=w4240, y=w4236) -> (x/y=w4244:dbl)
                    n2529 = Reshape Array(w4246, w4244, w4236) -> (w4245:u64[][])
                    n2530 = Transpose 2D Array(2D array=w4245) -> (transposed array=w4243:u64[][])
                    n2531 = for {
                      tunnel: w4243 -> [w4248] mode=indexing
                      tunnel: [w4247] -> w4237 mode=indexing
                      tunnel: w4239 -> [w4249]
                      workers-P: _ -> [_]
                      n2532 = call "downsample 1D array - U64.vi"("Ave N"=w4249, "Array In"=w4248) -> ("Array Out"=w4247:u64[])  [unwired: 1 in]
                    }
                    n2533 = Transpose 2D Array(2D array=w4237) -> (transposed array=w4242:u64[][])
                    n2534 = Divide(x=w4240, y=w4239) -> (x/y=w4241:dbl)
                    n2535 = Reshape Array(w4242, w4241) -> (w4238:u64[])
                  }
                }
                n2536 = case shown="False" w4166 {
                  tunnel: w4226 -> [w4258 w4270]
                  tunnel: [w4258 w4262] -> w4222
                  tunnel: "Save ave N" -> [_ w4263]
                  tunnel: w4217 -> [_ w4261]
                  frame False {
                  }
                  frame True {
                    n2537 = Array Size(array=w4270) -> (size(s)=w4264:i32)
                    n2538 = Array Size(array=w4261) -> (size(s)=w4260:i32)
                    n2539 = Divide(x=w4264, y=w4260) -> (x/y=w4268:dbl)
                    n2540 = Reshape Array(w4270, w4268, w4260) -> (w4269:i16[][])
                    n2541 = Transpose 2D Array(2D array=w4269) -> (transposed array=w4267:i16[][])
                    n2542 = for {
                      tunnel: w4267 -> [w4273] mode=indexing
                      tunnel: [w4272] -> w4259 mode=indexing
                      tunnel: w4263 -> [w4271]
                      workers-P: _ -> [_]
                      n2543 = call "downsample 1D array - I16.vi"("Ave N"=w4271, "Array In"=w4273) -> ("Array Out"=w4272:i16[])  [unwired: 1 out]
                    }
                    n2544 = Transpose 2D Array(2D array=w4259) -> (transposed array=w4266:i16[][])
                    n2545 = Divide(x=w4264, y=w4263) -> (x/y=w4265:dbl)
                    n2546 = Reshape Array(w4266, w4265) -> (w4262:i16[])
                  }
                }
                n2547 = Index Array(array=w4188, index=1) -> (element=w4191:waveform(dbl))
                n2548 = Index Array(array=w4188, index=0) -> (element=w4193:waveform(dbl))
                n2549 = Unbundle By Name(w4191) -> ("Y"=w4195:dbl[])
                n2550 = Unbundle By Name(w4193) -> ("Y"=w4203:dbl[])
                n2551 = case "Write trap pos. data" shown="True" w4169 {
                  tunnel: w4168 -> [_ w4251]
                  tunnel: w4164 -> [_ w4250]
                  frame False {
                  }
                  frame True {
                    n2552 = Write to Binary File(file (use dialog)=w4251, data=w4250, 5:FALSE ("prepend array or string size? (T)"), 9:T24."big-endian, network order" ("byte order (0:big-endian, network order)")) -> ()  [unwired: 1 in, 4 out]
                  }
                }
                n2553 = Write to Binary File(file (use dialog)=w4229, data=w4222, 5:FALSE ("prepend array or string size? (T)"), 9:T24."big-endian, network order" ("byte order (0:big-endian, network order)")) -> ()  [unwired: 1 in, 4 out]
                n2554 = feedback #33(w4195) -> (w4197:dbl[])
                n2555 = Build Array (concatenate)(w4197, w4195) -> (w4196:dbl[])
                n2556 = Select(t=w4195, s=w4171, f=w4196) -> (s? t:f=w4181:dbl[])
                n2557 = feedback-in #33(w4181) -> ()
                n2558 = feedback #34(w4203) -> (w4216:dbl[])
                n2559 = Build Array (concatenate)(w4216, w4203) -> (w4215:dbl[])
                n2560 = Select(t=w4203, s=w4171, f=w4215) -> (s? t:f=w4190:dbl[])
                n2561 = feedback-in #34(w4190) -> ()
                n2562 = Divide(x=w4230, y=w4231) -> (x/y=w4233:dbl)
                n2563 = Multiply(x=w4233, y=100.0) -> (x*y=w4232:dbl)
                n2564 = Build Array(w4190, w4181) -> (→"Saved APD":dbl[][])
                n2565 = Array Size(array=w4190) -> (size(s)=w4208:i32)
                n2566 = Unbundle By Name(w4210) -> ("Y"=w4214:dbl[])
                n2567 = Subtract(x=w4208, y="N pts to average") -> (x-y=w4184:i32)
                n2568 = Multiply(x="N pts to average", y=u16 2) -> (x*y=w4185:u16)
                n2569 = Subtract(x=w4208, y=w4185) -> (x-y=w4183:i32)
                n2570 = feedback #35(w4214) -> (w4213:dbl[])
                n2571 = Build Array (concatenate)(w4213, w4214) -> (w4212:dbl[])
                n2572 = Select(t=w4214, s=w4171, f=w4212) -> (s? t:f=w4211:dbl[])
                "Trap Delta Graph" <- w4211
                n2573 = feedback-in #35(w4211) -> ()
                n2574 = Array Subset(array=w4190, index=w4184, length="N pts to average") -> (w4207:dbl[])
                n2575 = Array Subset(array=w4190, index=w4183, length="N pts to average") -> (w4206:dbl[])
                n2576 = Array Subset(array=w4181, index=w4184, length="N pts to average") -> (w4187:dbl[])
                n2577 = Array Subset(array=w4181, index=w4183, length="N pts to average") -> (w4186:dbl[])
                n2578 = call <vilib>:"Mean.vi"("X"=w4207) -> ("mean"=w4205:dbl)  [unwired: 1 out]
                n2579 = call <vilib>:"Mean.vi"("X"=w4187) -> ("mean"=w4180:dbl)  [unwired: 1 out]
                n2580 = call <vilib>:"Mean.vi"("X"=w4206) -> ("mean"=w4204:dbl)  [unwired: 1 out]
                n2581 = call <vilib>:"Mean.vi"("X"=w4186) -> ("mean"=w4179:dbl)  [unwired: 1 out]
                n2582 = Subtract(x=w4180, y=w4179) -> (x-y=w4170:dbl)
                "Delta Fl. 2" <- w4170
                n2583 = Subtract(x=w4205, y=w4204) -> (x-y=w4202:dbl)
                "Delta Fl. 1" <- w4202
                n2584 = Initialize Array(w4202, 1 ("dimension size")) -> (w4199:dbl[])
                n2585 = Initialize Array(w4170, 1 ("dimension size")) -> (w4176:dbl[])
                n2586 = feedback #36(w4199) -> (w4200:dbl[])
                n2587 = Build Array (concatenate)(w4200, w4199) -> (w4198:dbl[])
                n2588 = feedback #37(w4176) -> (w4177:dbl[])
                n2589 = Build Array (concatenate)(w4177, w4176) -> (w4175:dbl[])
                n2590 = Select(t=w4199, s=w4171, f=w4198) -> (s? t:f=w4174:dbl[])
                n2591 = feedback-in #36(w4174) -> ()
                n2592 = Select(t=w4176, s=w4171, f=w4175) -> (s? t:f=w4173:dbl[])
                n2593 = feedback-in #37(w4173) -> ()
                n2594 = Build Array(w4174, w4173) -> (→"Save APD Deriv":dbl[][])
              }
            }
            "Progress" <- w4147
            "Progress 2" <- w4147
          }
        }
      }
    }
    n2595 = Bundle By Name(cluster=w2843, "Green FB Ch 0"=w2842, "Green FB Ch 1"=w2841) -> (w2821:T47)
    "Green FB Signals (V)" <- w2821
    n2596 = Unbundle By Name(w2821) -> ("Green FB Ch 2"=→"Green FB Plot":dbl)
    n2597 = local read "wait to reset values"() -> (w2912:bool)
    n2598 = Not(x=w2910) -> (.not. x?=w2913:bool)
    n2599 = And(x=w2913, y=w2912) -> (x .and. y?=w2914:bool)
    n2600 = case "Part of MCL raster scanning: returns to initial positions after scan done" shown="True" w2914 {
      tunnel: w2627 -> [w3689 w3696]
      tunnel: [w3689 w3695] -> w2916
      tunnel: w2626 -> [w3688 w3694]
      tunnel: [w3688 w3693] -> w2911
      frame False {
      }
      frame True {
        w3704 = 10.0 ("y")
        w3703 = 32767.0 ("y")
        # "to return scan values\nafter a synchronous \nAOM scan"
        n2601 = local read "AO2"() -> (w3697:dbl)
        n2602 = local read "AO1"() -> (w3698:dbl)
        n2603 = local write "wait to reset values"(FALSE ("wait to reset values")) -> ()
        n2604 = Multiply(x=w3698, y=w3703) -> (x*y=w3700:dbl)
        n2605 = Multiply(x=w3697, y=w3703) -> (x*y=w3702:dbl)
        n2606 = Divide(x=w3700, y=w3704) -> (x/y=w3699:dbl)
        n2607 = Divide(x=w3702, y=w3704) -> (x/y=w3701:dbl)
        n2608 = To Word Integer(number=w3699) -> (16bit integer=w3705:i16)
        n2609 = To Word Integer(number=w3701) -> (16bit integer=w3706:i16)
        n2610 = local read "Total Counts (ticks)"() -> (w3690:u32)
        n2611 = xnode "Read/Write Control"("FPGA VI Reference In"=w3696, "error in"=w3694, "AO1"=w3705, "AO2"=w3706, "MCL count"=w3690) -> ("FPGA VI Reference Out"=w3695:T19, "error out"=w3693:errorcluster)
        n2612 = local read "Scan Range (V)\n(of steps)"() -> (w3691:dbl)
        n2613 = property on="Scan Range (V)\n(of steps)" class="DigNum (strict)"("Val(Sgnl)"=w3691) -> ()  [unwired: 2 in, 2 out]
      }
    }
    n2614 = node-c288() -> ()  [unwired: 2 out]
  }
  n2615 = node-c288(w81) -> ()  [unwired: 1 out]
  n2616 = node-c288(w83) -> ()  [unwired: 1 out]
  n2617 = node-c288(w68) -> ()  [unwired: 1 out]
  n2618 = VISA Close(VISA resource name=w72, error in (no error)=w71) -> (error out=w120:errorcluster)
  n2619 = call <vilib>:"Simple Error Handler.vi"("error in (no error)"=w120) -> ()  [unwired: 1 in, 8 out]
  n2620 = node-c288(w79) -> ()  [unwired: 1 out]
  n2621 = node-c288(w164) -> ()  [unwired: 1 out]
  n2622 = flat-sequence {
    tunnel: w258 -> [w4277]
    tunnel: w260 -> [w4278]
    tunnel: [w4276] -> w239
    tunnel: [w4275] -> w238
    tunnel: w220 -> [_]
    tunnel: w172 -> [_]
    tunnel: w85 -> [_]
    tunnel: w239 -> [w4279]
    tunnel: w238 -> [w4280]
    frame #0 {
      w4274 = FALSE ("AI to FIFO")
      n2623 = xnode "Read/Write Control"("FPGA VI Reference In"=w4278, "error in"=w4277, "AI to FIFO"=w4274, "APD to FIFO"=w4274) -> ("FPGA VI Reference Out"=w4276:T19, "error out"=w4275:errorcluster)
    }
    frame #1 {
      n2624 = xnode "Close FPGA VI Reference"("FPGA VI Reference In"=w4279, "error in"=w4280) -> ("error out"=→"error out":errorcluster)
    }
  }
